vi "Read system_index.vi"(11 "Heater in":refnum<class "Heater_v2.lvclass">) -> (2 "system_index":i32, 3 "Heater out":refnum<class "Heater_v2.lvclass">)   [LabVIEW 2019, in "Heater_v2.lvclass"]
uses:
  Heater_v2.lvclass
  Heater_v2.lvclass/Heater_v2.ctl
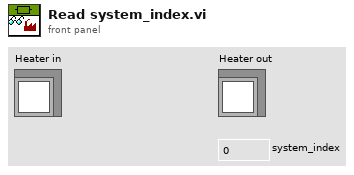
[diagram p1: front panel]
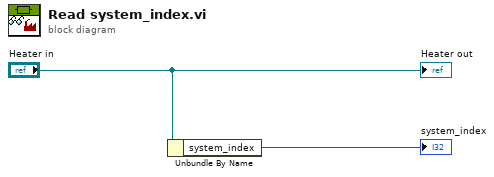
[diagram p0: block diagram]
diagram:
  n1 = Unbundle By Name("Heater in") -> ("system_index"=→"system_index":i32)
  "Heater out" <- "Heater in"
